vi "Read_weights.vi"(0 "sensor":u16(ring) items=["sensor1", "sensor 2", "sensor 3"]) -> (1 "weights 1":dbl[][](array[numeric]), 2 "weights 2":dbl[][](array[numeric]))   [LabVIEW 2009]
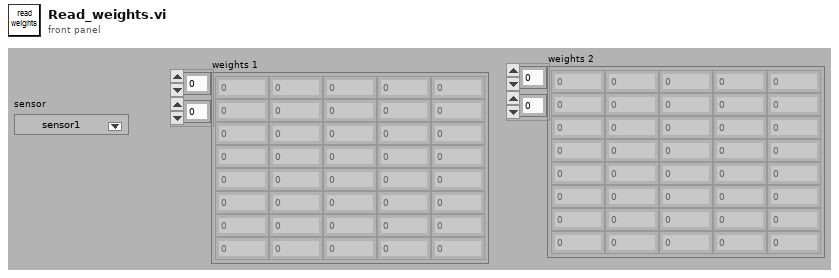
[diagram p1: front panel]
types:
  T1 = enum16{"open", "replace", "create", "open or create", "replace or create", "replace or create with confirmation"}
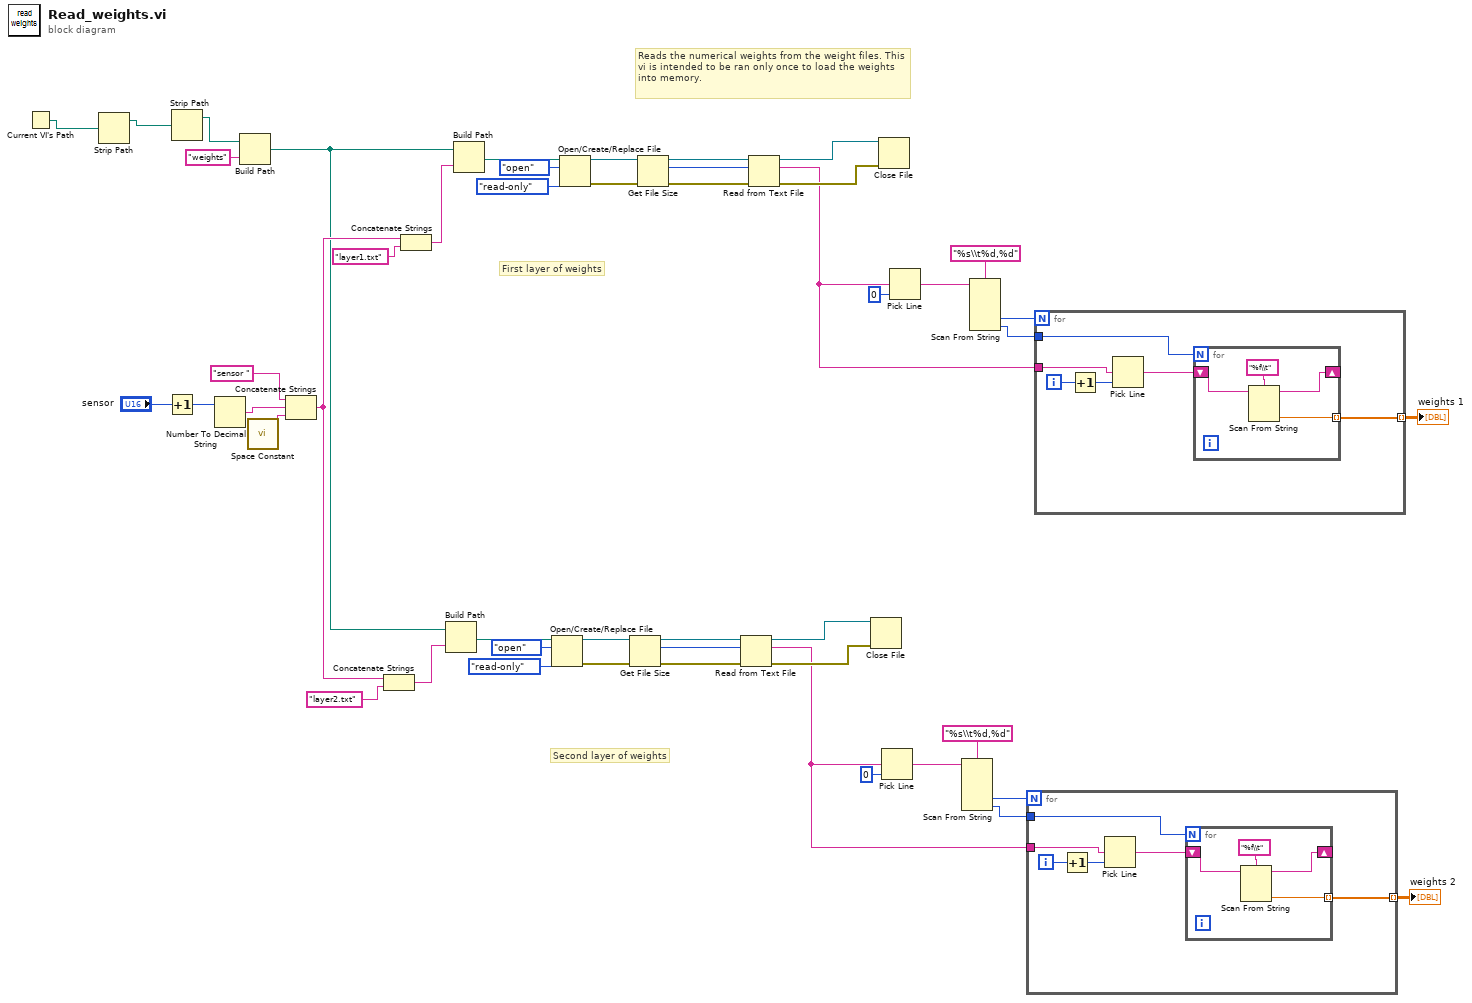
[diagram p0: block diagram]
diagram:
  # "Second layer of weights"
  # "First layer of weights"
  # "Reads the numerical weights from the weight files. This vi is intended to be ran only once to load the weights into memory."
  n1 = Current VI's Path() -> (path=w2:path)
  n2 = Strip Path(path=w2) -> (stripped path=w1:path)  [unwired: 1 out]
  n3 = Increment(x="sensor") -> (x+1=w14:u16)
  n4 = Strip Path(path=w1) -> (stripped path=w5:path)  [unwired: 1 out]
  n5 = Number To Decimal String(number=w14) -> (decimal integer string=w13:string)  [unwired: 1 in]
  n6 = Build Path(base path=w5, name or relative path="weights") -> (appended path=w3:path)
  n7 = call <vilib>:"Space Constant.vi"() -> ("String"=w11:string)
  n8 = Concatenate Strings("sensor ", w13, w11) -> (w8:string)
  n9 = Concatenate Strings(w8, "layer2.txt") -> (w9:string)
  n10 = Concatenate Strings(w8, "layer1.txt") -> (w6:string)
  n11 = Build Path(base path=w3, name or relative path=w9) -> (appended path=w33:path)
  n12 = Build Path(base path=w3, name or relative path=w6) -> (appended path=w49:path)
  n13 = Open/Create/Replace File(file path (use dialog)=w33, operation (0:open)=T1."open", access (0:read/write)=enum16{"read/write", "read-only", "write-only"}."read-only") -> (refnum out=w30:refnum<file>, error out=w29:errorcluster)  [unwired: 3 in, 1 out]
  n14 = Open/Create/Replace File(file path (use dialog)=w49, operation (0:open)=T1."open", access (0:read/write)=enum16{"read/write", "read-only", "write-only"}."read-only") -> (refnum out=w46:refnum<file>, error out=w45:errorcluster)  [unwired: 3 in, 1 out]
  n15 = Get File Size(file=w30, error in=w29) -> (refnum out=w28:refnum<file>, size (in bytes)=w24:i64, 0:w27:errorcluster)
  n16 = Get File Size(file=w46, error in=w45) -> (refnum out=w44:refnum<file>, size (in bytes)=w40:i64, 0:w43:errorcluster)
  n17 = Read from Text File(file (use dialog)=w28, count=w24, error in=w27) -> (refnum out=w26:refnum<file>, text=w19:string, error out=w25:errorcluster)  [unwired: 1 in, 1 out]
  n18 = Read from Text File(file (use dialog)=w44, count=w40, error in=w43) -> (refnum out=w42:refnum<file>, text=w35:string, error out=w41:errorcluster)  [unwired: 1 in, 1 out]
  n19 = Close File(refnum=w26, error in=w25) -> ()  [unwired: 2 out]
  n20 = Close File(refnum=w42, error in=w41) -> ()  [unwired: 2 out]
  n21 = Pick Line(multi-line string=w19, line index=0) -> (output string=w22:string)  [unwired: 1 in]
  n22 = Pick Line(multi-line string=w35, line index=0) -> (output string=w38:string)  [unwired: 1 in]
  n23 = Scan From String(format string="%s\\t%d,%d", input string=w22) -> (output 2=w20:i32, output 3=w18:i32)  [unwired: 6 in, 3 out]
  n24 = Scan From String(format string="%s\\t%d,%d", input string=w38) -> (output 2=w36:i32, output 3=w34:i32)  [unwired: 6 in, 3 out]
  n25 = for {
    N: w20 -> [_]
    tunnel: w19 -> [w53]
    tunnel: w18 -> [w52]
    tunnel: [w50] -> w16 mode=indexing
    i -> [w55]
    n26 = Increment(x=w55) -> (x+1=w54:i32)
    n27 = Pick Line(multi-line string=w53, line index=w54) -> (output string=w51:string)  [unwired: 1 in]
    n28 = for {
      N: w52 -> [_]
      tunnel: [w57] -> w50 mode=indexing
      shift-right: [w56] -> _
      shift-left: w51 -> [w58]
      n29 = Scan From String(format string="%f\\t", input string=w58) -> (remaining string=w56:string, output 1=w57:dbl)  [unwired: 3 in, 2 out]
    }
  }
  "weights 2" <- w16
  n30 = for {
    N: w36 -> [_]
    tunnel: w35 -> [w63]
    tunnel: w34 -> [w62]
    tunnel: [w60] -> w17 mode=indexing
    i -> [w65]
    n31 = Increment(x=w65) -> (x+1=w64:i32)
    n32 = Pick Line(multi-line string=w63, line index=w64) -> (output string=w61:string)  [unwired: 1 in]
    n33 = for {
      N: w62 -> [_]
      tunnel: [w67] -> w60 mode=indexing
      shift-right: [w66] -> _
      shift-left: w61 -> [w68]
      n34 = Scan From String(format string="%f\\t", input string=w68) -> (remaining string=w66:string, output 1=w67:dbl)  [unwired: 3 in, 2 out]
    }
  }
  "weights 1" <- w17
